vi "Ramsete_Diff_DO_Eng.vi"(5 "WheelBase-Feet":dbl=2.0, 6 "Gyro-Deg":dbl, 7 "Reset":bool, 8 "RightDist-Feet":dbl, 9 "LeftDist-Feet":dbl, 10 "TRAJ_STATE":T5={"TimeSeconds"=0.0, "Velocity"=0.0, "Acceleration"=0.0, "POSE"={"TRANSLATION"={"X"=0.0, "Y"=0.0}, "ROTATION"={"VALUE"=0.0, "COS"=1.0, "SIN"=0.0}}, "Curvature"=0.0} {"POSE"."ROTATION"."SIN" format="%13.4f"; "POSE"."ROTATION"."COS" format="%13.4f"; "POSE"."ROTATION"."VALUE" format="%13.4f"; "POSE"."TRANSLATION"."Y" format="%14.3f"; "POSE"."TRANSLATION"."X" format="%14.3f"}, 11 "inRAMSETE":T1={"B"=2.0, "Zeta"=0.7, "poseTolerance"={"TRANSLATION"={"X"=0.0, "Y"=0.0}, "ROTATION"={"VALUE"=0.0, "COS"=1.0, "SIN"=0.0}}, "poseError"={"TRANSLATION"={"X"=0.0, "Y"=0.0}, "ROTATION"={"VALUE"=0.0, "COS"=1.0, "SIN"=0.0}}, "Enabled"=TRUE} {"poseError"."ROTATION"."SIN" format="%13.4f"; "poseError"."ROTATION"."COS" format="%13.4f"; "poseError"."ROTATION"."VALUE" format="%13.4f"; "poseError"."TRANSLATION"."Y" format="%14.3f"; "poseError"."TRANSLATION"."X" format="%14.3f"; "poseTolerance"."ROTATION"."SIN" format="%13.4f"; "poseTolerance"."ROTATION"."COS" format="%13.4f"; "poseTolerance"."ROTATION"."VALUE" format="%13.4f"; "poseTolerance"."TRANSLATION"."Y" format="%14.3f"; "poseTolerance"."TRANSLATION"."X" format="%14.3f"; "Zeta" format="%12.3f"; "B" format="%12.3f"}) -> (0 "AtReference":bool, 1 "RightVelDmd-FT/SEC":dbl, 2 "LeftVelDmd-FT/SEC":dbl, 3 "outRAMSETE":T1={"B"=2.0, "Zeta"=0.7, "poseTolerance"={"TRANSLATION"={"X"=0.0, "Y"=0.0}, "ROTATION"={"VALUE"=0.0, "COS"=1.0, "SIN"=0.0}}, "poseError"={"TRANSLATION"={"X"=0.0, "Y"=0.0}, "ROTATION"={"VALUE"=0.0, "COS"=1.0, "SIN"=0.0}}, "Enabled"=TRUE} {"poseError"."ROTATION"."SIN" format="%13.4f"; "poseError"."ROTATION"."COS" format="%13.4f"; "poseError"."ROTATION"."VALUE" format="%13.4f"; "poseError"."TRANSLATION"."Y" format="%14.3f"; "poseError"."TRANSLATION"."X" format="%14.3f"; "poseTolerance"."ROTATION"."SIN" format="%13.4f"; "poseTolerance"."ROTATION"."COS" format="%13.4f"; "poseTolerance"."ROTATION"."VALUE" format="%13.4f"; "poseTolerance"."TRANSLATION"."Y" format="%14.3f"; "poseTolerance"."TRANSLATION"."X" format="%14.3f"; "Zeta" format="%12.3f"; "B" format="%12.3f"}, 4 "CurrentRelativePose_ENG":T2 {"ROTATION"."SIN" format="%13.4f"; "ROTATION"."COS" format="%13.4f"; "ROTATION"."VALUE" format="%13.4f"; "TRANSLATION"."Y" format="%14.3f"; "TRANSLATION"."X" format="%14.3f"})   [LabVIEW 2019]
doc: "This is a convience function that takes sensor data, and trajectory demands, then performs differential drive odometry, and executes ramsete control to output wheel speed demands.\n\nAll input and output units are Feet, Degrees. The TrajectoryState units are Meters,Radians\n\nParameters:\n - InRamsete - Ramsete data structure\n - LeftDist - Left wheel distance\n - RightDist - Right wheel distance\n - Gyro - Robot gyro reading\n - Reset - Reset's the internal saved robot position, left / right distance, and gyro readings. This should be set true at the beginning of executing a trajectory.\n - TrajState - The desired trajectory state\n - WheelBase - The robot wheel base\n\nReturns:\n - outRamsete - Updated Ramsete data structure\n - AtReference - TRUE when robot position is withing tolerance\n - CurrentPose - Current robot Pose\n - LeftVelDmd - Left wheel velocity demand (These demands are NOT normalized.)\n -RightVelDmd - Right wheel velocity demand (These demands are NOT normalized.)"
uses:
  Trajectory_Library.lvlib
  TypeDef/TRANSLATION2D.ctl
  TypeDef/ROTATION2D.ctl
  TypeDef/POSE2D.ctl
  TypeDef/TRAJ_STATE.ctl
  TypeDef/RAMSETE.ctl
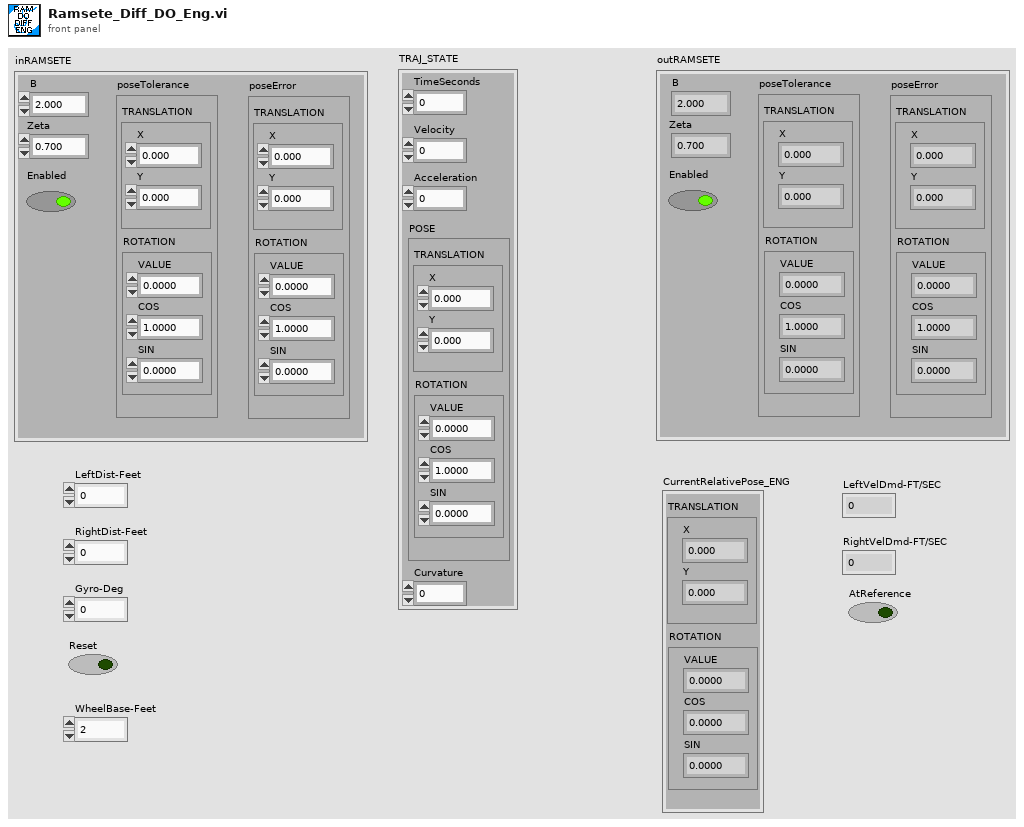
[diagram p1: front panel]
types:
  T1 = typedef "Trajectory_Library.lvlib/RAMSETE.ctl" = cluster{"B":dbl, "Zeta":dbl, "poseTolerance":T2, "poseError":T2, "Enabled":bool}
  T2 = typedef "Trajectory_Library.lvlib/POSE2D.ctl" = cluster{"TRANSLATION":T3, "ROTATION":T4}
  T3 = typedef "Trajectory_Library.lvlib/TRANSLATION2D.ctl" = cluster{"X":dbl, "Y":dbl}
  T4 = typedef "Trajectory_Library.lvlib/ROTATION2D.ctl" = cluster{"VALUE":dbl, "COS":dbl, "SIN":dbl}
  T5 = typedef "Trajectory_Library.lvlib/TRAJ_STATE.ctl" = cluster{"TimeSeconds":dbl, "Velocity":dbl, "Acceleration":dbl, "POSE":T2, "Curvature":dbl}
  T6 = typedef "Trajectory_Library.lvlib/DIFF_DRIVE_KINEMATICS.ctl" = cluster{"TrackWidth_Meters":dbl}
  T7 = typedef "Trajectory_Library.lvlib/CHASSIS_SPEEDS.ctl" = cluster{"vX":dbl, "vY":dbl, "vOmega":dbl}
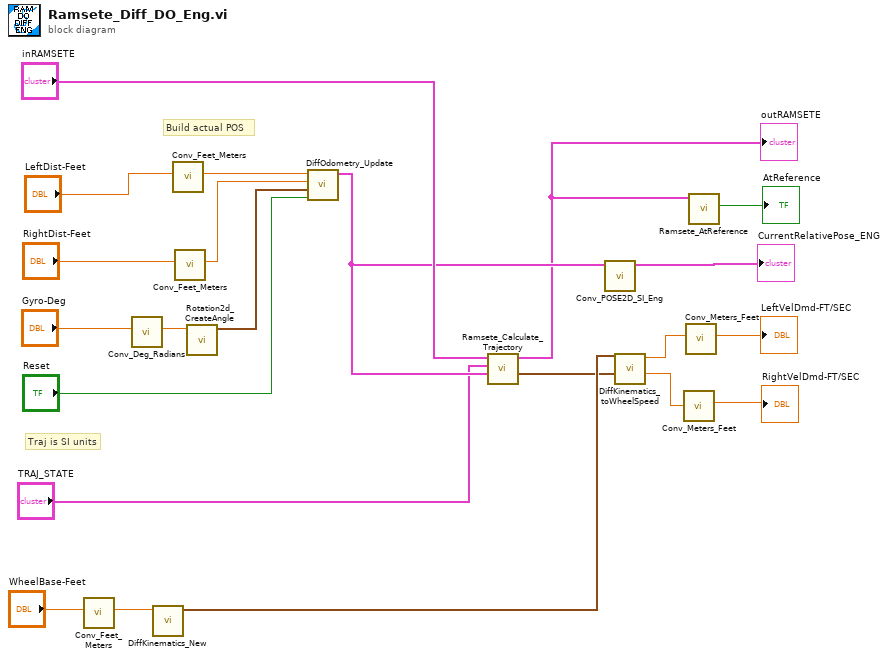
[diagram p0: block diagram]
diagram:
  # "Traj is SI units"
  # "Build actual POS"
  n1 = call "Conv_Feet_Meters.vi"("Feet"="WheelBase-Feet") -> ("Meters"=w10:dbl)  [unwired: 10 in]
  n2 = call "Conv_Deg_Radians.vi"("Degress"="Gyro-Deg") -> ("Radians"=w11:dbl)  [unwired: 10 in]
  n3 = call "DiffKinematics_New.vi"("TrackWidth_Meters"=w10) -> ("DIFF_DRIVE_KINEMATICS"=w9:T6)  [unwired: 10 in]
  n4 = call "Conv_Feet_Meters.vi"("Feet"="LeftDist-Feet") -> ("Meters"=w16:dbl)  [unwired: 10 in]
  n5 = call "Conv_Feet_Meters.vi"("Feet"="RightDist-Feet") -> ("Meters"=w17:dbl)  [unwired: 10 in]
  n6 = call "Rotation2d_CreateAngle.vi"("Angle"=w11) -> ("ROTATION"=w12:T4)  [unwired: 10 in]
  n7 = call "DiffOdometry_Update.vi"("Reset"="Reset", "Heading"=w12, "RightDistance"=w17, "LeftDistance"=w16) -> ("CurrentRelativePose"=w5:T2)  [unwired: 7 in]
  n8 = call "Ramsete_Calculate_Trajectory.vi"("CurrentPOSE"=w5, "TRAJ_STATE"="TRAJ_STATE", "inRAMSETE"="inRAMSETE") -> ("CHASSIS Speeds"=w3:T7, "outRAMSETE"=w1:T1)  [unwired: 7 in]
  "outRAMSETE" <- w1
  n9 = call "Conv_POSE2D_SI_Eng.vi"("Err Pose in SI"=w5) -> ("Err Pose out ENG"=→"CurrentRelativePose_ENG":T2)  [unwired: 10 in]
  n10 = call "DiffKinematics_toWheelSpeed.vi"("CHASSIS Speed"=w3, "DIFF_DRIVE_KINEMATICS"=w9) -> ("RightVelocity"=w19:dbl, "LeftVelocity"=w18:dbl)  [unwired: 8 in]
  n11 = call "Conv_Meters_Feet.vi"("Meters"=w19) -> ("Feet"=→"RightVelDmd-FT/SEC":dbl)  [unwired: 10 in]
  n12 = call "Conv_Meters_Feet.vi"("Meters"=w18) -> ("Feet"=→"LeftVelDmd-FT/SEC":dbl)  [unwired: 10 in]
  n13 = call "Ramsete_AtReference.vi"("RAMSETE"=w1) -> ("AtReference"=→"AtReference":bool)  [unwired: 10 in]
